vi "Create One Column Table HTML From Channel List.vi"(6 "Instance ID":string, 7 "engine configuration in":refnum<class "engine configuration.lvclass">, 8 "Node#":i32, 9 "Color":string="invis", 10 "Title":string, 11 "Channels":refnum<class "TBM channel.lvclass">[](array[class])) -> (2 "Table HTML":string, 3 "Channel and Node Pairs":T1[](array[typedef]))   [LabVIEW 2013, in "GraphViz Mapping Visualizer.lvlib"]
uses:
  GraphViz Mapping Visualizer.lvlib
  <vilib>/NI/Tag Bus Module Framework/channel/TBM channel.lvclass
  Channel to Port Pair.ctl
  <vilib>/NI/Module Execution Interface/Engine Configuration/engine configuration.lvclass
  <vilib>/NI/Tag Bus/tag/tag descriptor.lvclass/tag descriptor.ctl
  <vilib>/NI/Tag Bus/tag/read tag name.vi
  <vilib>/NI/Tag Bus/tag/tag descriptor.lvclass
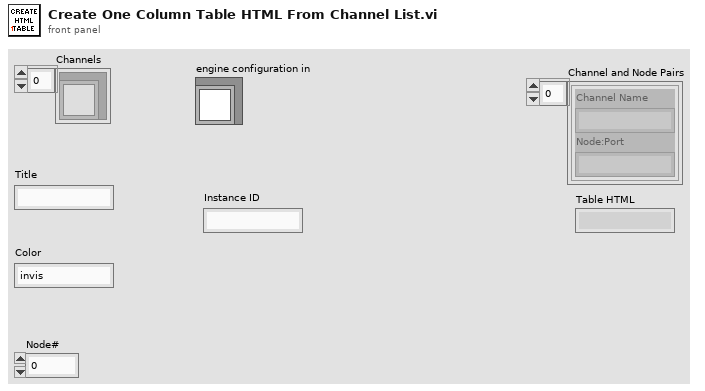
[diagram p1: front panel]
types:
  T1 = typedef "GraphViz Mapping Visualizer.lvlib/Channel to Port Pair.ctl" = cluster{"Channel Name":string, "Node:Port":string}
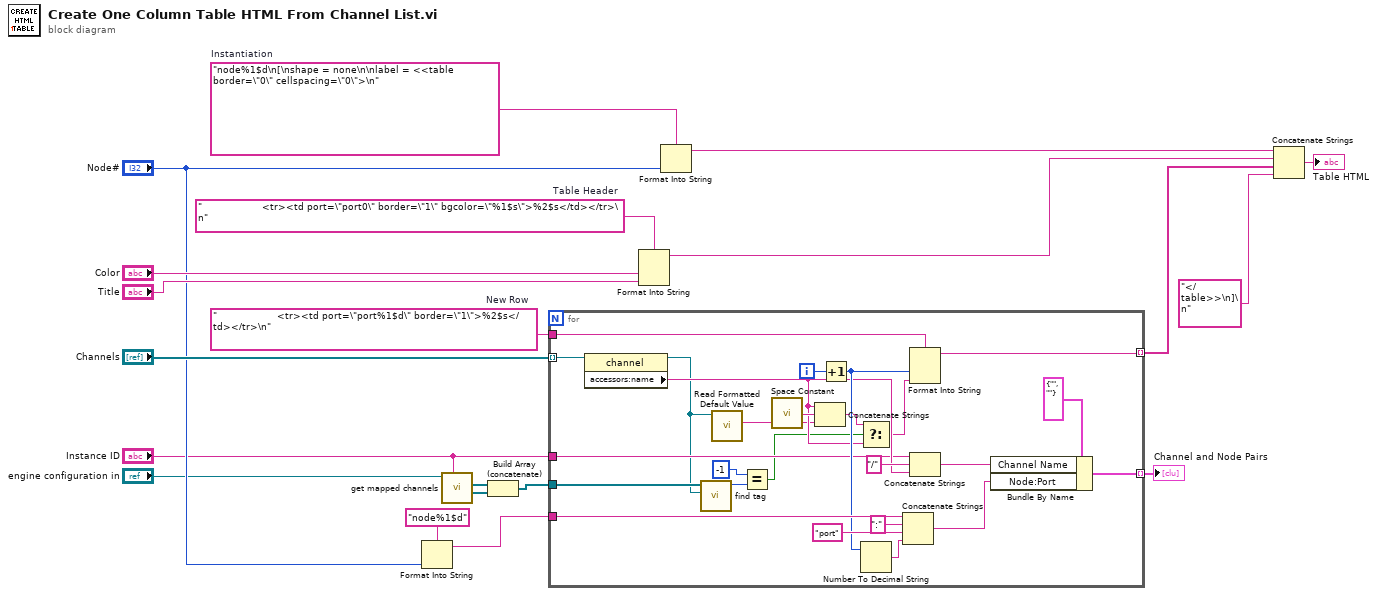
[diagram p0: block diagram]
diagram:
  w12 = "node%1$d\n[\nshape = none\n\nlabel = <<table border=\"0\" cellspacing=\"0\">\n"  # Instantiation
  w17 = "                    <tr><td port=\"port0\" border=\"1\" bgcolor=\"%1$s\">%2$s</td></tr>\n"  # Table Header
  w20 = "                    <tr><td port=\"port%1$d\" border=\"1\">%2$s</td></tr>\n"  # New Row
  n1 = Format Into String(format string="node%1$d", "Node#") -> (resulting string=w7:string)  [unwired: 2 in, 1 out]
  n2 = call <vilib>:"get mapped channels.vi"("owner"="Instance ID", "engine configuration in"="engine configuration in") -> ("write channels"=w2:refnum<class "TBM channel.lvclass">[], "read channels"=w3:refnum<class "TBM channel.lvclass">[])  [unwired: 5 in, 3 out]
  n3 = Build Array (concatenate)(w3, w2) -> (w1:refnum<class "TBM channel.lvclass">[])
  n4 = for {
    tunnel: "Channels" -> [w44] mode=indexing
    tunnel: [w43] -> w13 mode=indexing
    tunnel: w20 -> [w42]
    tunnel: w7 -> [w39]
    tunnel: "Instance ID" -> [w27]
    tunnel: [w32] -> w6 mode=indexing
    tunnel: w1 -> [w23]
    i -> [w45]
    n5 = property class="channel"(reference=w44) -> (reference out=w22:refnum<class "TBM channel.lvclass">, "accessors:name"=w29:string)  [unwired: 1 in, 1 out]
    n6 = call <vilib>:"find tag.vi"("tag"=w22, "tags in"=w23) -> ("index"=w25:i32)  [unwired: 9 in]
    n7 = call "Read Formatted Default Value.vi"("channel"=w22) -> ("Formatted Default"=w21:string)  [unwired: 9 in, 1 out]
    n8 = Equal?(x=-1, y=w25) -> (x = y?=w24:bool)
    n9 = call <vilib>:"Space Constant.vi"() -> ("String"=w31:string)
    n10 = Concatenate Strings(w29, w31, w21) -> (w30:string)
    n11 = Increment(x=w45) -> (x+1=w38:i32)
    n12 = Select(t=w30, s=w24, f=w29) -> (s? t:f=w28:string)
    n13 = Number To Decimal String(number=w38) -> (decimal integer string=w37:string)  [unwired: 1 in]
    n14 = Concatenate Strings(w39, ":" ("string"), "port" ("string"), w37) -> (w35:string)
    n15 = Format Into String(format string=w42, w38, w28) -> (resulting string=w43:string)  [unwired: 2 in, 1 out]
    n16 = Concatenate Strings(w27, "/", w29) -> (w33:string)
    n17 = Bundle By Name(cluster=T1 {"Channel Name"="", "Node:Port"=""} ("Channel to Port Pair"), "Channel Name"=w33, "Node:Port"=w35) -> (w32:T1)
  }
  "Channel and Node Pairs" <- w6
  n18 = Format Into String(format string=w17, "Color", "Title") -> (resulting string=w14:string)  [unwired: 2 in, 1 out]
  n19 = Format Into String(format string=w12, "Node#") -> (resulting string=w11:string)  [unwired: 2 in, 1 out]
  n20 = Concatenate Strings(w11, w14, w13, "</table>>\n]\n") -> (→"Table HTML":string)
